vi "Schreibe Tabelle.vi"(10 "Points":T3(array[cluster])) -> (2 "Table":T1(array[cluster]))   [LabVIEW 2017]
uses:
  AT901 API/Structures/Struct TransformationPoint.ctl
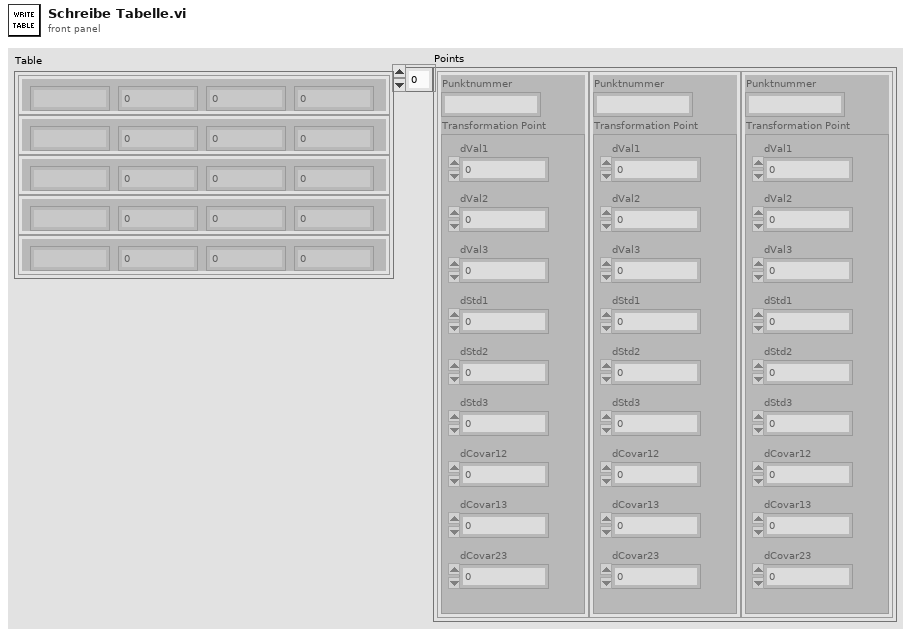
[diagram p1: front panel]
types:
  T1 = cluster{"X":dbl, "Y":dbl, "Z":dbl, "Punktnummer":string}[]
  T2 = typedef "Struct TransformationPoint.ctl" = cluster{"dVal1":dbl, "dVal2":dbl, "dVal3":dbl, "dStd1":dbl, "dStd2":dbl, "dStd3":dbl, "dCovar12":dbl, "dCovar13":dbl, "dCovar23":dbl}
  T3 = cluster{"Punktnummer":string, "Transformation Point":T2}[]
  T4 = cluster{"X":dbl, "Y":dbl, "Z":dbl, "Punktnummer":string}
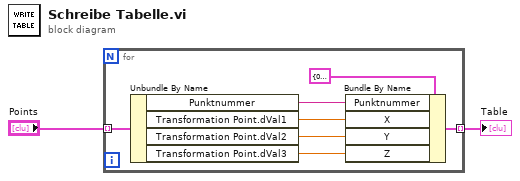
[diagram p0: block diagram]
diagram:
  n1 = for {
    tunnel: "Points" -> [w9] mode=indexing
    tunnel: [w8] -> w1 mode=indexing
    n2 = Unbundle By Name(w9) -> ("Punktnummer"=w6:string, "Transformation Point.dVal1"=w5:dbl, "Transformation Point.dVal2"=w4:dbl, "Transformation Point.dVal3"=w3:dbl)
    n3 = Bundle By Name(cluster=T4 {"X"=0.0, "Y"=0.0, "Z"=0.0, "Punktnummer"=""}, "Punktnummer"=w6, "X"=w5, "Y"=w4, "Z"=w3) -> (w8:T4)
  }
  "Table" <- w1
